vi "ScriptWireTunnels.vi"(8 "error in":errorcluster, 9 "i/o terminals":refnum<vi>[](array[refnum]), 10 "CaseStructure in":refnum<vi>, 11 "ControlTerminal in":refnum<vi>) -> (0 "error out":errorcluster)   [LabVIEW 2024]
uses:
  <vilib>/Utility/miscctls.llb/LVBoundsTypeDef.ctl
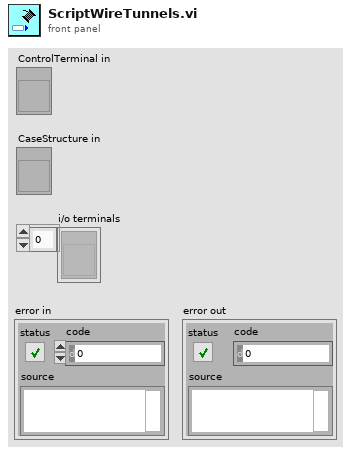
[diagram p1: front panel]
types:
  T1 = typedef "LVBoundsTypeDef.ctl" = cluster{"Width":u32, "Height":u32}
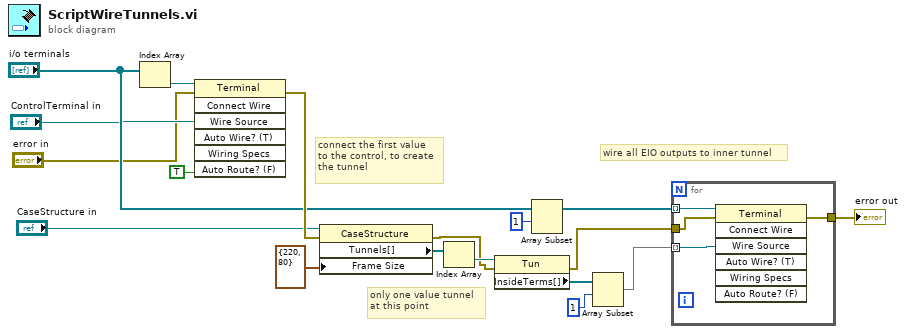
[diagram p0: block diagram]
diagram:
  # "connect the first value\nto the control, to create\nthe tunnel"
  # "wire all EIO outputs to inner tunnel"
  # "only one value tunnel\nat this point"
  n1 = Index Array(array="i/o terminals") -> (element=w15:refnum<vi>)  [unwired: 1 in]
  n2 = invoke on="Invoke Node" class="Terminal" method="Connect Wire"(reference=w15, error in="error in", "Wire Source"="ControlTerminal in", "Auto Route? (F)"=TRUE) -> (error out=w18:errorcluster)  [unwired: 3 in, 6 out]
  n3 = property class="CaseStructure"(reference="CaseStructure in", error in=w18, "Frame Size"=T1 {"Width"=220, "Height"=80}) -> (error out=w2:errorcluster, "Tunnels[]"=w12:refnum<vi>[])  [unwired: 1 out]
  n4 = Index Array(array=w12) -> (element=w14:refnum<vi>)  [unwired: 1 in]
  n5 = property class="Tun"(reference=w14, error in=w2) -> (error out=w1:errorcluster, "InsideTerms[]"=w7:refnum<vi>[])  [unwired: 1 out]
  n6 = Array Subset(array="i/o terminals", index=1) -> (w4:refnum<vi>[])  [unwired: 1 in]
  n7 = Array Subset(array=w7, index=1) -> (w5:refnum<vi>[])  [unwired: 1 in]
  n8 = for {
    tunnel: w5 -> [w21] mode=indexing
    tunnel: w4 -> [w19] mode=indexing
    tunnel: [w22] -> w16
    tunnel: w1 -> [w20]
    n9 = invoke on="Invoke Node" class="Terminal" method="Connect Wire"(reference=w19, error in=w20, "Wire Source"=w21) -> (error out=w22:errorcluster)  [unwired: 4 in, 6 out]
  }
  "error out" <- w16
